vi "SetAllSides.vi"(8 "error in (no error)":errorcluster, 10 "RoomSides":T1[](array[typedef]), 11 "Room in":refnum<class "Room.lvclass">) -> (0 "error out":errorcluster, 3 "Room out":refnum<class "Room.lvclass">)   [LabVIEW 2020, in "Room.lvclass"]
uses:
  Room.lvclass
  FactoryMethod/GoF_Example/NoParametrizedFactoryMethod/MazeGame/Private/TypeDef/RoomElement.ctl
  MazeSite/MazeSite.lvclass
  Direction.ctl
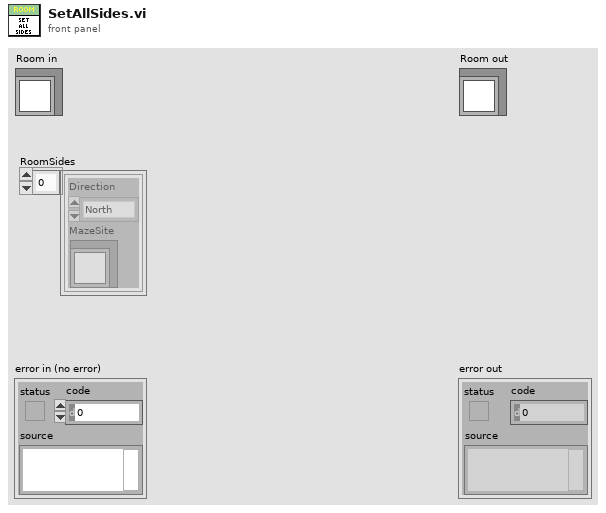
[diagram p1: front panel]
types:
  T1 = typedef "Room.lvclass/RoomElement.ctl" = cluster{"Direction":T2, "MazeSite":refnum<class "MazeSite.lvclass">}
  T2 = typedef "Direction.ctl" = enum32{"North", "South", "East", "West"}
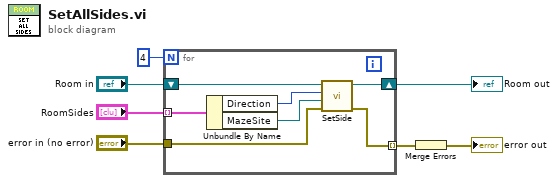
[diagram p0: block diagram]
diagram:
  n1 = for {
    N: 4 -> [_]
    shift-right: [w13] -> w1
    shift-left: "Room in" -> [w14]
    tunnel: "RoomSides" -> [w12] mode=indexing
    tunnel: "error in (no error)" -> [w9]
    tunnel: [w8] -> w3 mode=indexing
    n2 = Unbundle By Name(w12) -> ("Direction"=w11:T2, "MazeSite"=w10:refnum<class "MazeSite.lvclass">)
    n3 = call "SetSide.vi"("error in (no error)"=w9, "MazeSite"=w10, "Direction"=w11, "Room in"=w14) -> ("error out"=w8:errorcluster, "Room out"=w13:refnum<class "Room.lvclass">)  [unwired: 6 in]
  }
  "Room out" <- w1
  n4 = Merge Errors(w3) -> (→"error out":errorcluster)
